vi "Main.vi"() -> ()   [LabVIEW 2014]
doc: "The boiler controller allows a user to start and shut down a boiler.\n\nUse the Reset, Start, and Light Pilot controls to sequentially start the boiler. \nUse the Fuel Control Valve to change the flow of fuel into the boiler. \nUse the Stop Boiler button to shut down the boiler. \nTo shut down the system or in the event of an emergency, use the Emergency Stop button to close the application completely."
uses:
  controls/MHL Data.ctl
  controls/MHL UI Data.ctl
  controls/MHL Status.ctl
  controls/MHL References.ctl
  controls/MHL Configuration.ctl
  support/Boiler System Globals.vi
  <vilib>/Utility/error.llb/Error Cluster From Error Code.vi
  <vilib>/ErrorRing/Error Ring.xnode
  support/Message Queue/Message Queue.lvlib
  support/User Event - Stop/User Event - Stop.lvlib
  Controller/Controller.lvlib
  Boiler/Boiler.lvlib
panel:
  in  "Fuel Control Valve":u32(slide) min=10 max=75 scale=10.0..75.0
  in  "Stop Boiler":bool
  in  "Light Pilot":bool
  out "Forced Draft Fan":bool
  out "Pilot":bool
  out "Pilot Gas Valve":bool
  out "Primary Fan":bool
  out "Status":string
  in  "Start":bool
  in  "Reset":bool
  in  "Emergency Stop":bool
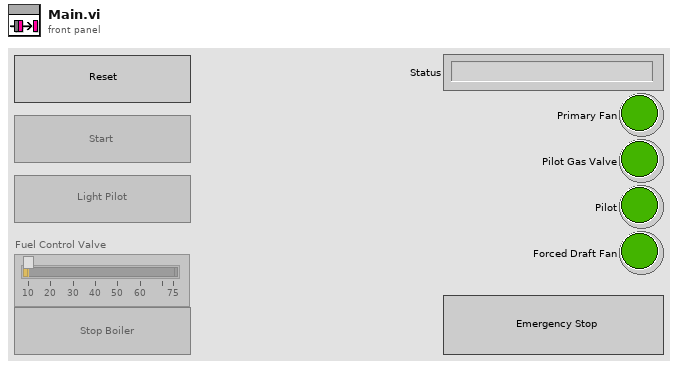
[diagram p1: front panel]
types:
  T1 = typedef "MHL Data.ctl" = cluster{"MHL User Interface Data":T2, "MHL References":T4, "MHL Configuration":T5}
  T2 = typedef "MHL UI Data.ctl" = cluster{"Status":string, "Fuel Control Valve":u32, "Primary Fan":bool, "Pilot Gas Valve":bool, "Pilot":bool, "Forced Draft Fan":bool, "MHL Status":T3}
  T3 = typedef "MHL Status.ctl" = enum16{"Lockout", "Ready", "Pre-Purge", "Pre-Purge Complete", "Pilot On", "Boiler Running", "Shutdown", "Purge"}
  T4 = typedef "MHL References.ctl" = cluster{"Reset Ref":refnum<vi>, "Start Ref":refnum<vi>, "Light Pilot Ref":refnum<vi>, "Stop Boiler Ref":refnum<vi>, "Fuel Control Valve Ref":refnum<vi>}
  T5 = typedef "MHL Configuration.ctl" = cluster{"Fuel Control Valve Maximum":dbl, "Fuel Control Valve Minimum":dbl}
  T6 = typedef "Configuration Data.ctl" = cluster{"MHL Configuration":T5, "Controller Configuration":T7, "Boiler Configuration":T8}
  T7 = typedef "Controller.lvlib/Controller Configuration.ctl" = cluster{"Purge Time":u32, "Flame Threshold":u32}
  T8 = typedef "Boiler.lvlib/Boiler Configuration.ctl" = cluster{"Pilot Increment (ms)":u32, "Pilot Decrement (ms)":u32}
  T9 = typedef "Notifiers.ctl" = cluster{"Handshake":refnum<notifier>, "Flame Level":refnum<notifier>, "Controller Exit":refnum<notifier>, "Boiler Exit":refnum<notifier>}
  T10 = typedef "Message Queue.lvlib/All Message Queues.ctl" = cluster{"MHL":refnum<queue>, "Boiler Controller":refnum<queue>, "Boiler":refnum<queue>}
  T11 = enum16{"open", "replace", "create", "open or create", "replace or create", "replace or create with confirmation"}
  T12 = enum32{"invalid app kind", "Development System", "Run Time System", "Student Edition", "Embedded LabVIEW", "Evaluation", "Custom"}
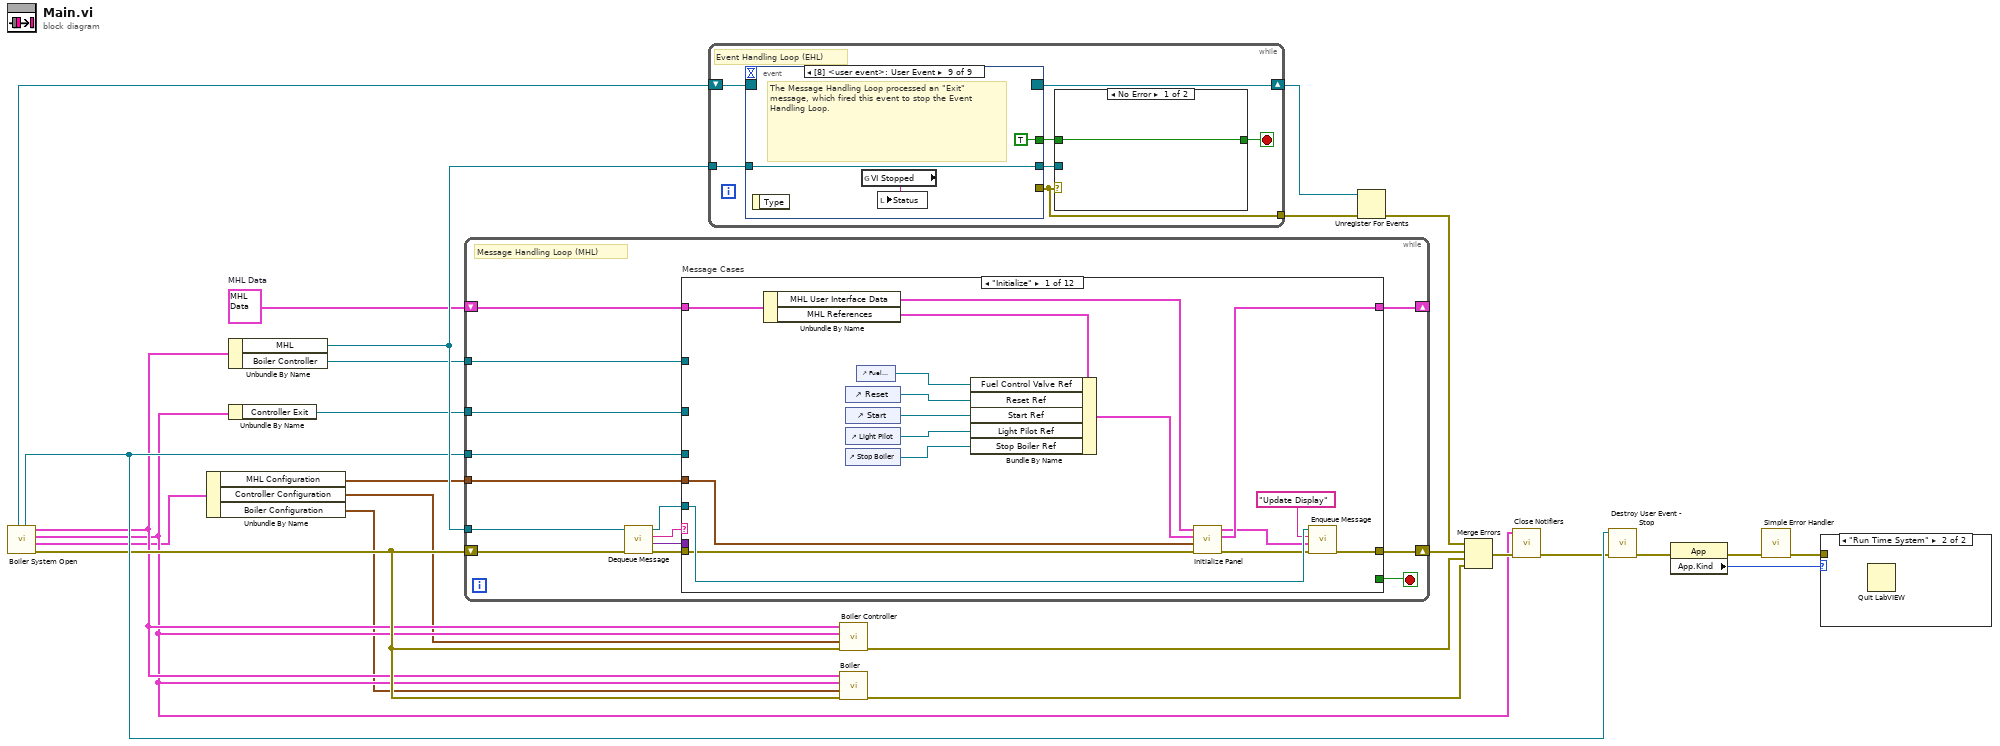
[diagram p0: block diagram]
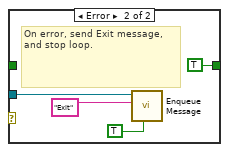
[diagram p3: hidden frame]
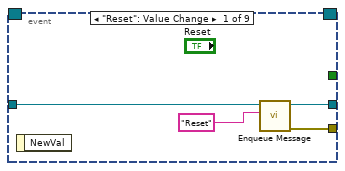
[diagram p4: hidden frame]
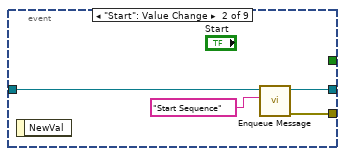
[diagram p5: hidden frame]
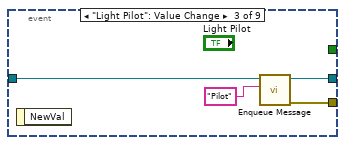
[diagram p6: hidden frame]
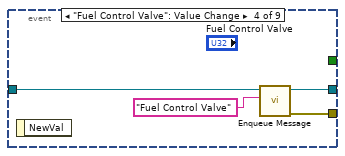
[diagram p7: hidden frame]
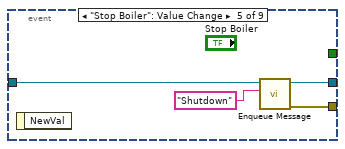
[diagram p8: hidden frame]
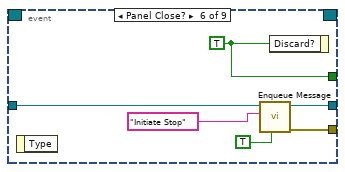
[diagram p9: hidden frame]
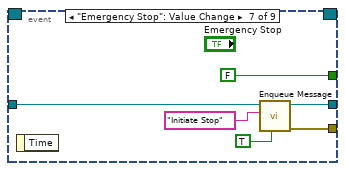
[diagram p10: hidden frame]
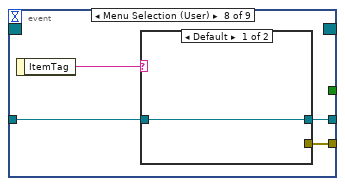
[diagram p11: hidden frame]
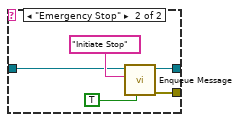
[diagram p12: hidden frame]
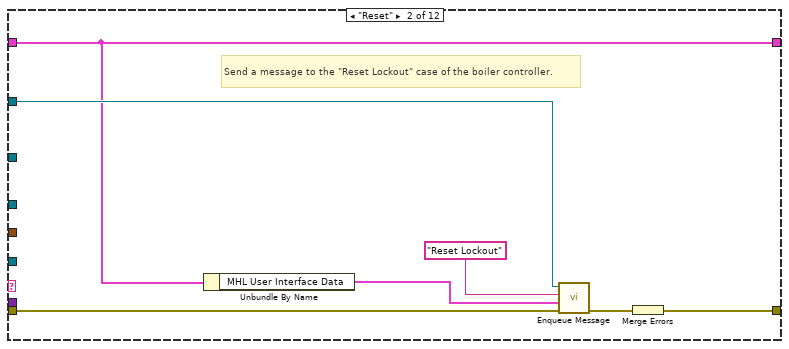
[diagram p13: hidden frame]
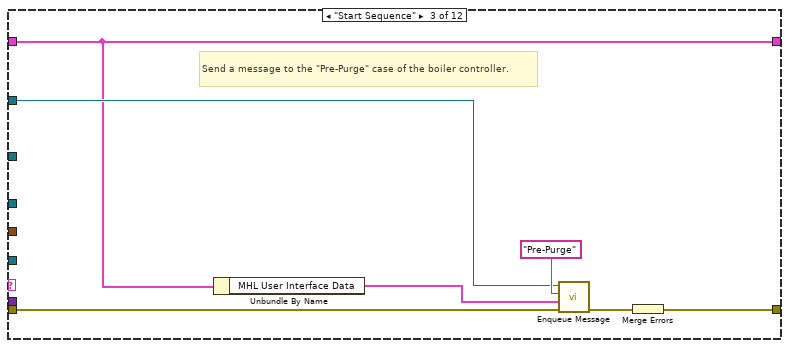
[diagram p14: hidden frame]
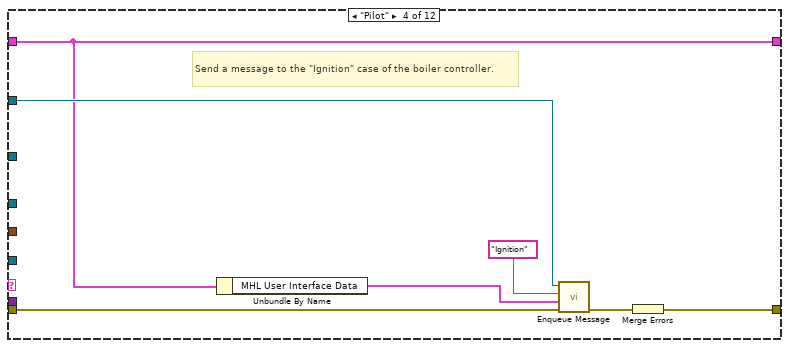
[diagram p15: hidden frame]
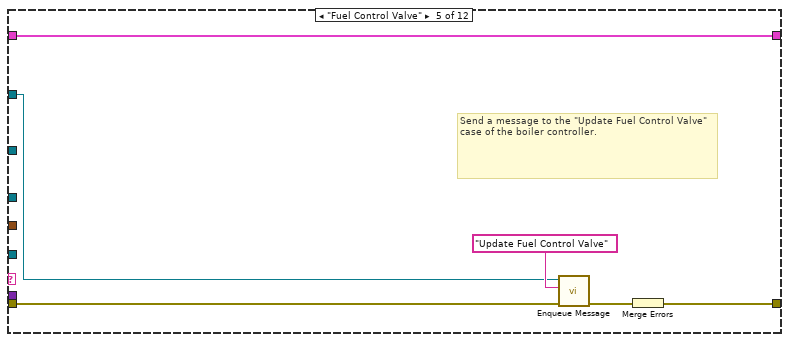
[diagram p16: hidden frame]
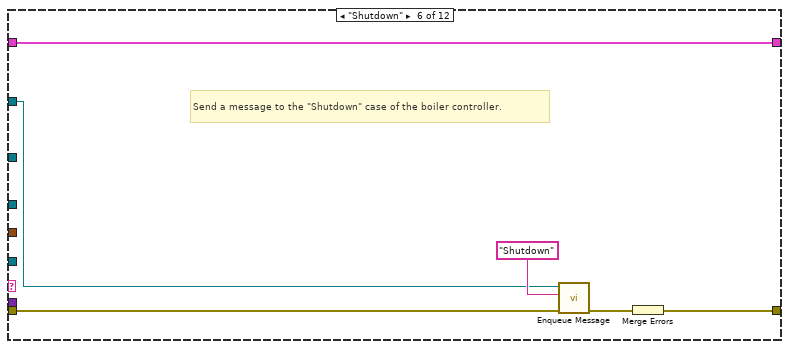
[diagram p17: hidden frame]
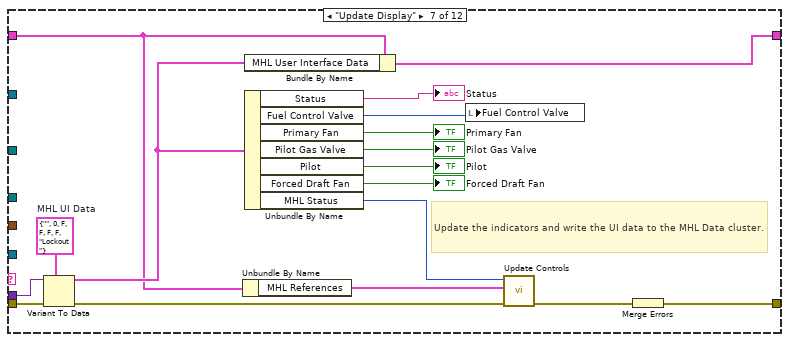
[diagram p18: hidden frame]
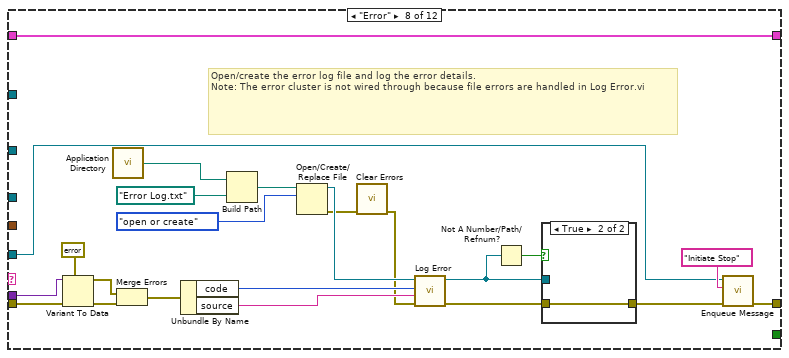
[diagram p19: hidden frame]
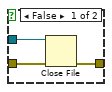
[diagram p20: hidden frame]
diagram:
  w19 = T1 {"MHL User Interface Data"={"Status"="", "Fuel Control Valve"=0, "Primary Fan"=FALSE, "Pilot Gas Valve"=FALSE, "Pilot"=FALSE, "Forced Draft Fan"=FALSE, "MHL Status"=enum."Lockout"}, "MHL References"={"Reset Ref"=refnum, "Start Ref"=refnum, "Light Pilot Ref"=refnum, "Stop Boiler Ref"=refnum, "Fuel Control Valve Ref"=refnum}, "MHL Configuration"={"Fuel Control Valve Maximum"=0.0, "Fuel Control Valve Minimum"=0.0}}  # MHL Data
  n1 = call "Boiler System Open.vi"() -> ("error out"=w10:errorcluster, "Configuration Data"=w4:T6, "Notifiers"=w5:T9, "Message Queues"=w9:T10, "User Event - Stop"=w12:refnum<user-event>, "Stop Event Registration Refnum"=w13:refnum<event-registration>)  [unwired: 6 in]
  n2 = Unbundle By Name(w4) -> ("MHL Configuration"=w3:T5, "Controller Configuration"=w2:T7, "Boiler Configuration"=w1:T8)
  n3 = Unbundle By Name(w9) -> ("MHL"=w24:refnum<queue>, "Boiler Controller"=w17:refnum<queue>)
  n4 = Unbundle By Name(w5) -> ("Controller Exit"=w11:refnum<notifier>)
  n5 = while {
    tunnel: w24 -> [w29]
    shift-right: [w38] -> _
    shift-left: w19 -> [w39]
    tunnel: w12 -> [w35]
    shift-right: [w36] -> w25
    shift-left: w10 -> [w34]
    tunnel: w17 -> [w28]
    tunnel: w11 -> [w27]
    tunnel: w3 -> [w26]
    stop <- w37 stop-if-true
    # "Message Handling Loop (MHL)"
    n6 = call "Dequeue Message.vi"("error in (no error)"=w34, "Message Queue"=w29) -> ("error out"=w33:errorcluster, "Message Data"=w31:variant, "Message"=w32:string, "dup Message Queue"=w30:refnum<queue>)  [unwired: 6 in]
    n7 = case "Message Cases" shown="\"Initialize\"" w32 {
      selector: w32 -> [_ _ _ _ _ _ _ _ _ _ _ w167]
      tunnel: w30 -> [w49 _ _ _ _ _ _ w115 w136 w143 w165 _]
      tunnel: w33 -> [w43 w62 w69 w76 w78 w87 w105 w113 w141 w145 w158 _]
      tunnel: [w50 w63 w70 w77 w83 w88 w106 w111 w138 w144 w161 w166] -> w36
      tunnel: w39 -> [w51 w58 w65 w72 w79 w89 w91 w129 w140 w149 w164 w168]
      tunnel: [w41 w58 w65 w72 w79 w89 w95 w129 w140 w149 w164 w168] -> w38
      tunnel: [_ _ _ _ _ _ _ _ _ _ TRUE _] -> w37
      tunnel: w31 -> [_ _ _ _ _ _ w104 w112 _ _ _ _]
      tunnel: w35 -> [_ _ _ _ _ _ _ _ _ _ w160 _]
      tunnel: w28 -> [_ w59 w66 w73 w80 w84 _ _ w137 _ _ _]
      tunnel: w27 -> [_ _ _ _ _ _ _ _ _ w142 _ _]
      tunnel: w26 -> [w47 _ _ _ _ _ _ _ _ _ _ _]
      frame "Initialize" {
        n8 = Unbundle By Name(w51) -> ("MHL User Interface Data"=w44:T2, "MHL References"=w45:T4)
        n9 = control-ref of="Reset"() -> (w53:refnum<vi>)
        n10 = control-ref of="Start"() -> (w54:refnum<vi>)
        n11 = control-ref of="Light Pilot"() -> (w55:refnum<vi>)
        n12 = control-ref of="Stop Boiler"() -> (w56:refnum<vi>)
        n13 = control-ref of="Fuel Control Valve"() -> (w52:refnum<vi>)
        n14 = Bundle By Name(cluster=w45, "Fuel Control Valve Ref"=w52, "Reset Ref"=w53, "Start Ref"=w54, "Light Pilot Ref"=w55, "Stop Boiler Ref"=w56) -> (w46:T4)
        n15 = call "Initialize Panel.vi"("error in"=w43, "MHL Configuration"=w47, "MHL References"=w46, "MHL UI Data in"=w44) -> ("error out"=w42:errorcluster, "MHL Data out"=w41:T1, "MHL UI Data out"=w40:T2)  [unwired: 5 in]
        n16 = call "Enqueue Message.vi"("error in (no error)"=w42, "Message Data"=w40, "Message"="Update Display", "Message Queue"=w49) -> ("error out"=w50:errorcluster)  [unwired: 6 in, 1 out]
      }
      frame "Reset" {
        # "Send a message to the \"Reset Lockout\" case of the boiler controller."
        n17 = Unbundle By Name(w58) -> ("MHL User Interface Data"=w57:T2)
        n18 = call "Enqueue Message.vi"("error in (no error)"=w62, "Message Data"=w57, "Message"="Reset Lockout", "Message Queue"=w59) -> ("error out"=w61:errorcluster)  [unwired: 6 in, 1 out]
        n19 = Merge Errors(w61) -> (w63:errorcluster)
      }
      frame "Start Sequence" {
        # "Send a message to the \"Pre-Purge\" case of the boiler controller."
        n20 = Unbundle By Name(w65) -> ("MHL User Interface Data"=w64:T2)
        n21 = call "Enqueue Message.vi"("error in (no error)"=w69, "Message Data"=w64, "Message"="Pre-Purge", "Message Queue"=w66) -> ("error out"=w68:errorcluster)  [unwired: 6 in, 1 out]
        n22 = Merge Errors(w68) -> (w70:errorcluster)
      }
      frame "Pilot" {
        # "Send a message to the \"Ignition\" case of the boiler controller."
        n23 = Unbundle By Name(w72) -> ("MHL User Interface Data"=w71:T2)
        n24 = call "Enqueue Message.vi"("error in (no error)"=w76, "Message Data"=w71, "Message"="Ignition", "Message Queue"=w73) -> ("error out"=w75:errorcluster)  [unwired: 6 in, 1 out]
        n25 = Merge Errors(w75) -> (w77:errorcluster)
      }
      frame "Fuel Control Valve" {
        # "Send a message to the \"Update Fuel Control Valve\" case of the boiler controller."
        n26 = call "Enqueue Message.vi"("error in (no error)"=w78, "Message"="Update Fuel Control Valve", "Message Queue"=w80) -> ("error out"=w82:errorcluster)  [unwired: 7 in, 1 out]
        n27 = Merge Errors(w82) -> (w83:errorcluster)
      }
      frame "Shutdown" {
        # "Send a message to the \"Shutdown\" case of the boiler controller."
        n28 = call "Enqueue Message.vi"("error in (no error)"=w87, "Message"="Shutdown", "Message Queue"=w84) -> ("error out"=w86:errorcluster)  [unwired: 7 in, 1 out]
        n29 = Merge Errors(w86) -> (w88:errorcluster)
      }
      frame "Update Display" {
        w103 = T2 {"Status"="", "Fuel Control Valve"=0, "Primary Fan"=FALSE, "Pilot Gas Valve"=FALSE, "Pilot"=FALSE, "Forced Draft Fan"=FALSE, "MHL Status"=enum."Lockout"}  # MHL UI Data
        # "Update the indicators and write the UI data to the MHL Data cluster."
        n30 = Variant To Data(error in=w105, type=w103, Variant=w104) -> (data=w96:T2, error out=w94:errorcluster)
        n31 = Unbundle By Name(w91) -> ("MHL References"=w90:T4)
        n32 = Bundle By Name(cluster=w91, "MHL User Interface Data"=w96) -> (w95:T1)
        n33 = Unbundle By Name(w96) -> ("Status"=→"Status":string, "Fuel Control Valve"=w101:u32, "Primary Fan"=→"Primary Fan":bool, "Pilot Gas Valve"=→"Pilot Gas Valve":bool, "Pilot"=→"Pilot":bool, "Forced Draft Fan"=→"Forced Draft Fan":bool, "MHL Status"=w92:T3)
        n34 = local write "Fuel Control Valve"(w101) -> ()
        n35 = call "Update Controls.vi"("error in"=w94, "MHL References"=w90, "MHL Status"=w92) -> ("error out"=w93:errorcluster)  [unwired: 8 in]
        n36 = Merge Errors(w93) -> (w106:errorcluster)
      }
      frame "Error" {
        # "Open/create the error log file and log the error details.\nNote: The error cluster is not wired through because file errors are handled in Log Error.vi"
        n37 = Variant To Data(error in=w113, type=errorcluster {"status"=FALSE, "code"=0, "source"=""} ("error out"), Variant=w112) -> (data=w125:errorcluster, error out=w126:errorcluster)
        n38 = call <vilib>:"Application Directory.vi"() -> ("Application Directory"=w123:path)
        n39 = Merge Errors(w125, w126) -> (w124:errorcluster)
        n40 = Unbundle By Name(w124) -> ("code"=w118:i32, "source"=w117:string)
        n41 = Build Path(base path=w123, name or relative path=path "Error Log.txt") -> (appended path=w122:path)
        n42 = Open/Create/Replace File(file path (use dialog)=w122, operation (0:open)=T11."open or create") -> (refnum out=w120:refnum<file>, error out=w108:errorcluster)  [unwired: 4 in, 1 out]
        n43 = call <vilib>:"Clear Errors.vi"("error in (no error)"=w108) -> ("error out"=w107:errorcluster)  [unwired: 5 in, 1 out]
        n44 = call "Log Error.vi"("error in"=w107, "Source"=w117, "Code"=w118, "Error Log Refnum In"=w120) -> ("error out"=w119:errorcluster, "Error Log Refnum Out"=w110:refnum<file>)  [unwired: 6 in]
        n45 = Not A Number/Path/Refnum?(number/path/refnum=w110) -> (NaN/Path/Refnum?=w109:bool)
        n46 = case shown="True" w109 {
          tunnel: w119 -> [w132 w133]
          tunnel: w110 -> [w131 _]
          tunnel: [w130 w133] -> w116
          frame False {
            n47 = Close File(refnum=w131, error in=w132) -> (error out=w130:errorcluster)  [unwired: 1 out]
          }
          frame True {
          }
        }
        n48 = call "Enqueue Message.vi"("error in (no error)"=w116, "Message"="Initiate Stop", "Message Queue"=w115) -> ("error out"=w111:errorcluster)  [unwired: 7 in, 1 out]
      }
      frame "Initiate Stop" {
        # "When stopping, first send a message to stop the boiler controller. Then wait for the boiler and boiler controller to exit."
        n49 = call "Enqueue Message.vi"("error in (no error)"=w141, "Message"="Exit", "Message Queue"=w137) -> ("error out"=w139:errorcluster)  [unwired: 7 in, 1 out]
        n50 = call "Enqueue Message.vi"("error in (no error)"=w139, "Message"="Wait on Boiler Exit", "Message Queue"=w136) -> ("error out"=w138:errorcluster)  [unwired: 7 in, 1 out]
      }
      frame "Wait on Boiler Exit" {
        # "Monitor the boiler controller to determine if it has completed its Exit. Wait 10 milliseconds for the boiler controller to respond. \nIf the notification does not occur, then enqueue another Wait on Boiler Exit message.\nIf the notification occurs, then exit the Message Handling Loop."
        n51 = Wait on Notification(notifier=w142, timeout in ms (-1)=10, error in (no error)=w145) -> (timed out?=w147:bool, error out=w146:errorcluster)  [unwired: 1 in, 2 out]
        n52 = case shown="True" w147 {
          tunnel: w146 -> [w153 w157]
          tunnel: w143 -> [w152 w155]
          tunnel: [w150 w156] -> w144
          frame False {
            n53 = call "Enqueue Message.vi"("error in (no error)"=w153, "Message"="Exit", "Message Queue"=w152) -> ("error out"=w150:errorcluster)  [unwired: 7 in, 1 out]
          }
          frame True {
            n54 = call "Enqueue Message.vi"("error in (no error)"=w157, "Message"="Wait on Boiler Exit", "Message Queue"=w155) -> ("error out"=w156:errorcluster)  [unwired: 7 in, 1 out]
          }
        }
      }
      frame "Exit" {
        # "Stop the VI"
        # "Release the message queue reference"
        n55 = call "Fire User Event - Stop.vi"("User Event - Stop"=w160) -> ("error out"=w159:errorcluster)  [unwired: 10 in]
        n56 = Release Queue(queue=w165, error in (no error)=w158) -> (error out=w162:errorcluster)  [unwired: 1 in, 2 out]
        n57 = Merge Errors(w159, w162) -> (w161:errorcluster)
      }
      frame Default {
        # "'Default' case only runs if there is a message that isn't defined in any of the other cases.  Output a programming error."
        n58 = xnode "Error Ring"("parameter 0"=w167) -> ("error out"=w166:errorcluster)
      }
    }
  }
  n59 = while {
    tunnel: w24 -> [w182]
    tunnel: [w178] -> w21
    shift-right: [w176] -> w20
    shift-left: w13 -> [w177]
    stop <- w180 stop-if-true
    # "Event Handling Loop (EHL)"
    n60 = event shown="[8] <user event>: User Event" {
      selector: w177 -> [_ _ _ _ _ _ _ _ _]
      dyn-events: [_ _ _ _ _ _ _ _ _] -> w176
      timeout: _ -> [_ _ _ _ _ _ _ _ _]
      tunnel: [_ _ _ _ _ w213 FALSE ("Discard?") _ TRUE ("Discard?")] -> w181
      tunnel: w182 -> [w191 w195 w199 w203 w207 w212 w219 w222 w232]
      tunnel: [w190 w193 w197 w201 w205 w211 w218 w220 _] -> w178
      tunnel: [w189 w194 w198 w202 w206 w210 w216 w221 w232] -> w179
      event "Reset": Value Change {
        n61 = event-data() -> ()  [unwired: 1 in, 1 out]
        n62 = call "Enqueue Message.vi"("Message"="Reset", "Message Queue"=w191) -> ("error out"=w190:errorcluster, "dup Message Queue"=w189:refnum<queue>)  [unwired: 8 in]
      }
      event "Start": Value Change {
        n63 = event-data() -> ()  [unwired: 1 in, 1 out]
        n64 = call "Enqueue Message.vi"("Message"="Start Sequence", "Message Queue"=w195) -> ("error out"=w193:errorcluster, "dup Message Queue"=w194:refnum<queue>)  [unwired: 8 in]
      }
      event "Light Pilot": Value Change {
        n65 = event-data() -> ()  [unwired: 1 in, 1 out]
        n66 = call "Enqueue Message.vi"("Message"="Pilot", "Message Queue"=w199) -> ("error out"=w197:errorcluster, "dup Message Queue"=w198:refnum<queue>)  [unwired: 8 in]
      }
      event "Fuel Control Valve": Value Change {
        n67 = event-data() -> ()  [unwired: 1 in, 1 out]
        n68 = call "Enqueue Message.vi"("Message"="Fuel Control Valve", "Message Queue"=w203) -> ("error out"=w201:errorcluster, "dup Message Queue"=w202:refnum<queue>)  [unwired: 8 in]
      }
      event "Stop Boiler": Value Change {
        n69 = event-data() -> ()  [unwired: 1 in, 1 out]
        n70 = call "Enqueue Message.vi"("Message"="Shutdown", "Message Queue"=w207) -> ("error out"=w205:errorcluster, "dup Message Queue"=w206:refnum<queue>)  [unwired: 8 in]
      }
      event Panel Close? {
        w213 = TRUE ("Discard?")
        n71 = event-data() -> ()  [unwired: 1 in, 1 out]
        n72 = call "Enqueue Message.vi"("Priority Message? (F)"=TRUE, "Message"="Initiate Stop", "Message Queue"=w212) -> ("error out"=w211:errorcluster, "dup Message Queue"=w210:refnum<queue>)  [unwired: 7 in]
        n73 = event-data("Discard?"=w213) -> ()  [unwired: 1 in, 1 out]
      }
      event "Emergency Stop": Value Change {
        n74 = event-data() -> ()  [unwired: 1 in, 1 out]
        n75 = call "Enqueue Message.vi"("Priority Message? (F)"=TRUE, "Message"="Initiate Stop", "Message Queue"=w219) -> ("error out"=w218:errorcluster, "dup Message Queue"=w216:refnum<queue>)  [unwired: 7 in]
      }
      event Menu Selection (User) {
        n76 = event-data() -> ("ItemTag"=w223:string)  [unwired: 1 in]
        n77 = case shown="Default" w223 {
          tunnel: w222 -> [w224 w227]
          tunnel: [w224 w226] -> w221
          tunnel: [_ w225] -> w220
          frame Default {
          }
          frame "Emergency Stop" {
            n78 = call "Enqueue Message.vi"("Priority Message? (F)"=TRUE, "Message"="Initiate Stop", "Message Queue"=w227) -> ("error out"=w225:errorcluster, "dup Message Queue"=w226:refnum<queue>)  [unwired: 7 in]
          }
        }
      }
      event User Event {
        # "The Message Handling Loop processed an \"Exit\" message, which fired this event to stop the Event Handling Loop."
        n79 = event-data() -> ()  [unwired: 1 in, 1 out]
        n80 = global read "Boiler System Globals.vi" "VI Stopped"() -> (w230:string)
        n81 = local write "Status"(w230) -> ()
      }
    }
    n82 = case shown="No Error" w178 {
      tunnel: [w183 TRUE ("Discard?")] -> w180
      tunnel: w181 -> [w183 _]
      tunnel: w179 -> [_ w186]
      frame No Error {
      }
      frame Error {
        # "On error, send Exit message, and stop loop."
        n83 = call "Enqueue Message.vi"("Priority Message? (F)"=TRUE, "Message"="Exit", "Message Queue"=w186) -> ()  [unwired: 7 in, 2 out]
      }
    }
  }
  n84 = call "Boiler Controller.vi"("error in"=w10, "Controller Configuration"=w2, "Notifiers"=w5, "Message Queues"=w9) -> ("error out"=w18:errorcluster)  [unwired: 7 in]
  n85 = call "Boiler.vi"("error in"=w10, "Boiler Configuration"=w1, "Notifiers"=w5, "Message Queues"=w9) -> ("error out"=w8:errorcluster)  [unwired: 7 in]
  n86 = Unregister For Events(event registration refnum=w20, error in=w21) -> (error out=w22:errorcluster)
  n87 = Merge Errors(w22, w25, w18, w8) -> (w7:errorcluster)
  n88 = call "Close Notifiers.vi"("error in"=w7, "Notifiers"=w5) -> ("error out"=w6:errorcluster)  [unwired: 9 in]
  n89 = call "Destroy User Event - Stop.vi"("error in (no error)"=w6, "User Event - Stop"=w12) -> ("error out"=w23:errorcluster)  [unwired: 9 in]
  n90 = property class="App"(error in=w23) -> (error out=w16:errorcluster, "App.Kind"=w15:T12)  [unwired: 1 in, 1 out]
  n91 = call <vilib>:"Simple Error Handler.vi"("error in (no error)"=w16) -> ("error out"=w14:errorcluster)  [unwired: 4 in, 4 out]
  n92 = case shown="\"Run Time System\"" w15 {
    tunnel: w14 -> [_ _]
    frame Default {
    }
    frame "Run Time System" {
      n93 = Quit LabVIEW() -> ()  [unwired: 1 in]
    }
  }
